vi "FlowOut.vi"() -> (0 "error out":errorcluster)   [LabVIEW 2019, in "MPC_Laser Marked.lvclass"]
uses:
  MPC_Laser Marked.lvclass
  Function/IO Folder/IO_VI/IOCtrl/Ctrl/DMC1000B_1 SelectOutput.ctl
  Function/IO Folder/IO_VI/IOCtrl/Ctrl/DMC1000B_1 SelectIn.ctl
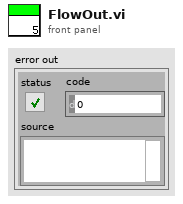
[diagram p1: front panel]
types:
  T1 = typedef "DMC1000B_1 SelectOutput.ctl" = enum16{"M_Out0預備", "M_OUT01蜂鳴器", "M_OUT02紅燈", "M_OUT03綠燈", "M_OUT04黃燈", "M_OUT05上頂固定位氣缸電磁閥", "M_OUT06到料阻擋氣缸電磁閥", "M_OUT07向前機台發出要料#1信號", "M_OUT08向前機台發出要料#2信號", "M_OUT09向後機台發出有料#3信號", "M_OUT10向後機台發出有料#4信號", "M_OUT11接駁台馬達啟動開/關", "M_OUT12接駁台馬達慢速", "M_OUT13抽風機開/關", "M_OUT14上視覺上光源", "M_OUT15DC吹風扇開/關", "M_OUT16Z軸煞車釋放", "M_OUT17", "M_OUT18", "M_OUT19", "M_OUT20", "M_OUT21", "M_OUT22", "M_OUT23", "M_OUT24", "M_OUT25第一軸SEVON1伺服使能信號", "M_OUT26第二軸SEVON2伺服使能信號", "M_OUT27第三軸SEVON3伺服使能信號"}
  T2 = typedef "DMC1000B_1 SelectIn.ctl" = enum16{"M_IN00預備", "M_IN01緊急急停檢測", "M_IN02啟動按鈕綠色", "M_IN03正壓氣壓檢知", "M_IN04安全門感知", "M_IN05接受前機台有料#1信號", "M_IN06接受前機台有料#2信號", "M_IN07接受後機台要料#3信號", "M_IN08接受後機台要料#4信號", "M_IN09軌道載板前進料到位檢知", "M_IN10到料阻擋氣缸上位檢知(阻擋位)", "M_IN11到料阻擋氣缸下位檢知(阻擋位)", "M_IN12上頂固定載板氣缸上位檢知", "M_IN13上頂固定載板氣缸下位檢知", "M_IN14軌道載板到位減速檢知", "M_IN15軌道載板到位檢知", "M_IN16軌道載板後出料檢知", "M_IN17", "M_IN18", "M_IN19", "M_IN20", "M_IN21第一軸準備輸入信號 RDY", "M_IN22第二軸準備輸入信號 RDY", "M_IN23第三軸準備輸入信號 RDY", "M_IN24", "M_IN25第一軸ALM+(  伺服警報輸出  )", "M_IN26第二軸ALM+(  伺服警報輸出  )", "M_IN27第三軸ALM+(  伺服警報輸出  )", "M_IN28", "M_IN29第一軸定位完成信號 INP", "M_IN30第二軸定位完成信號 INP", "M_IN31第三軸定位完成信號 INP", "M_IN32"}
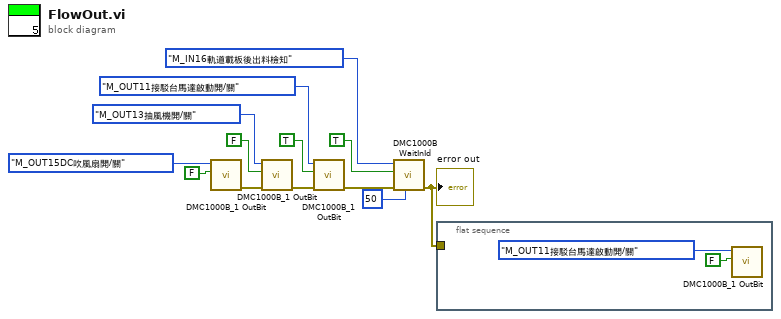
[diagram p0: block diagram]
diagram:
  n1 = call "DMC1000B_1 OutBit.vi"("BL"=FALSE, "IO_Output_1 Select"=DMC1000B_1_SelectOutput."M_OUT15DC吹風扇開/關") -> ("error out"=w8:errorcluster)  [unwired: 9 in]
  n2 = call "DMC1000B_1 OutBit.vi"("error in (no error)"=w8, "BL"=FALSE, "IO_Output_1 Select"=DMC1000B_1_SelectOutput."M_OUT13抽風機開/關") -> ("error out"=w13:errorcluster)  [unwired: 8 in]
  n3 = call "DMC1000B_1 OutBit.vi"("error in (no error)"=w13, "BL"=TRUE, "IO_Output_1 Select"=DMC1000B_1_SelectOutput."M_OUT11接駁台馬達啟動開/關") -> ("error out"=w6:errorcluster)  [unwired: 8 in]
  n4 = call "DMC1000B WaitInId.vi"("time(0.1)"=50, "error in"=w6, "Status"=TRUE, "64IIN_4 Select"=DMC1000B_1_SelectIn."M_IN16軌道載板後出料檢知") -> ("error Out"=w7:errorcluster)  [unwired: 5 in, 2 out]
  "error out" <- w7
  n5 = flat-sequence {
    tunnel: w7 -> [_]
    frame #0 {
      n6 = call "DMC1000B_1 OutBit.vi"("BL"=FALSE, "IO_Output_1 Select"=DMC1000B_1_SelectOutput."M_OUT11接駁台馬達啟動開/關") -> ()  [unwired: 9 in, 1 out]
    }
  }
